vi "KG get pump_a.vi"(8 "Fehler (Eingang, kein Fehler)":errorcluster, 10 "pump":u32, 11 "VISA-Ressourcenname":refnum<visa-resource-name>) -> (0 "Fehler (Ausgang)":errorcluster, 1 "Kommando gesendet":string, 2 "A":dbl, 3 "VISA-Ressourcenname (Ausgang)":refnum<visa-resource-name>)   [LabVIEW 2020, in "Linearisierung v2.lvlib" / "Gasteiler.lvlib" / "HovaCAL_Interface.lvlib" / "KGN.lvlib" / "get.lvlib"]
uses:
  get.lvlib
  KGN.lvlib
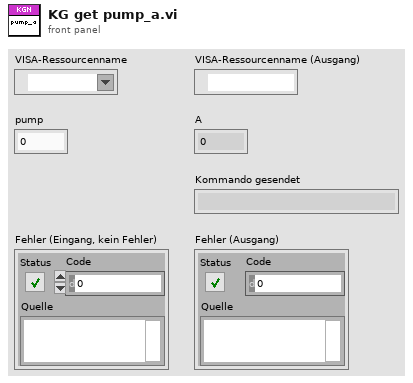
[diagram p1: front panel]
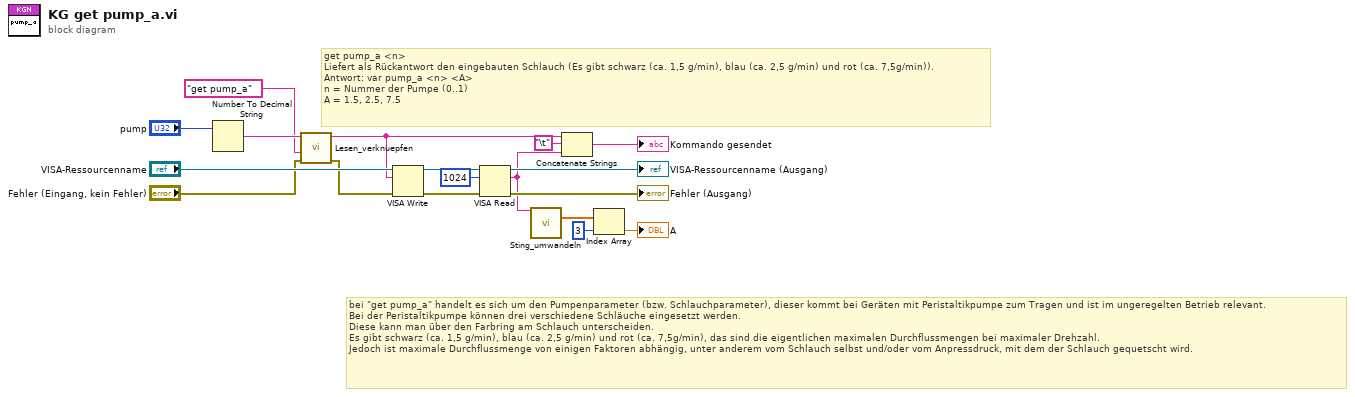
[diagram p0: block diagram]
diagram:
  # "bei \"get pump_a\" handelt es sich um den Pumpenparameter (bzw. Schlauchparameter), dieser kommt bei Geräten mit Peristaltikpumpe zum Tragen und ist im ungeregelten Betrieb relevant.\nBei der Peristaltikpumpe können drei verschiedene Schläuche eingesetzt werden.\nDiese kann man über den Farbring am Schlauch unterscheiden. \nEs gibt schwarz (ca. 1,5 g/min), blau (ca. 2,5 g/min) und rot (ca. 7,5g/min), das sind die eigentlichen maximalen Durchflussmengen bei maximaler Drehzahl.\nJedoch ist maximale Durchflussmenge von einigen Faktoren abhängig, unter anderem vom Schlauch selbst und/oder vom Anpressdruck, mit dem der Schlauch gequetscht wird."
  # "get pump_a <n>\nLiefert als Rückantwort den eingebauten Schlauch (Es gibt schwarz (ca. 1,5 g/min), blau (ca. 2,5 g/min) und rot (ca. 7,5g/min)).\nAntwort: var pump_a <n> <A>\nn = Nummer der Pumpe (0..1)\nA = 1.5, 2.5, 7.5"
  n1 = Number To Decimal String(number="pump") -> (decimal integer string=w8:string)  [unwired: 1 in]
  n2 = call "Lesen_verknuepfen.vi"("error in (no error)"="Fehler (Eingang, kein Fehler)", "Order"="get pump_a" ("Schreibpuffer"), "param"=w8) -> ("error out"=w10:errorcluster, "Verknüpfter String"=w9:string)  [unwired: 7 in]
  n3 = VISA Write(VISA resource name="VISA-Ressourcenname", write buffer=w9, error in (no error)=w10) -> (VISA resource name out=w18:refnum<visa-resource-name>, error out=w17:errorcluster)  [unwired: 1 out]
  n4 = VISA Read(VISA resource name=w18, byte count=u32 1024 ("Byte-Anzahl"), error in (no error)=w17) -> (VISA resource name out=→"VISA-Ressourcenname (Ausgang)":refnum<visa-resource-name>, read buffer=w2:string, error out=→"Fehler (Ausgang)":errorcluster)  [unwired: 1 out]
  n5 = call "Sting_umwandeln.vi"("Lesepuffer"=w2) -> ("Zahl array"=w5:dbl[])  [unwired: 8 in, 6 out]
  n6 = Concatenate Strings(w9, "\t", w2) -> (→"Kommando gesendet":string)
  n7 = Index Array(array=w5, index=3 ("Index")) -> (element=→"A":dbl)
